vi "Default MQTT Ack (Empty).vi"() -> (3 "No Ack":refnum<class "Ack.lvclass">)   [LabVIEW 2013]
uses:
  Ack.lvclass
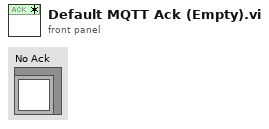
[diagram p1: front panel]
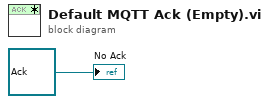
[diagram p0: block diagram]
diagram:
  "No Ack" <- refnum<class "Ack.lvclass"> refnum ("MQTT_Control_Packets.lvlib:Ack.lvclass")
